vi "Color Frame Data FGV.vi"(6 "Command":enum16{"Get", "Initialize"}(ring), 8 "error in (no error)":errorcluster, 10 "FrameDescription":T1) -> (0 "error out":errorcluster, 2 "Byte Array":u8[](array[numeric]))   [LabVIEW 2014]
uses:
  controls/FrameDescription.ctl
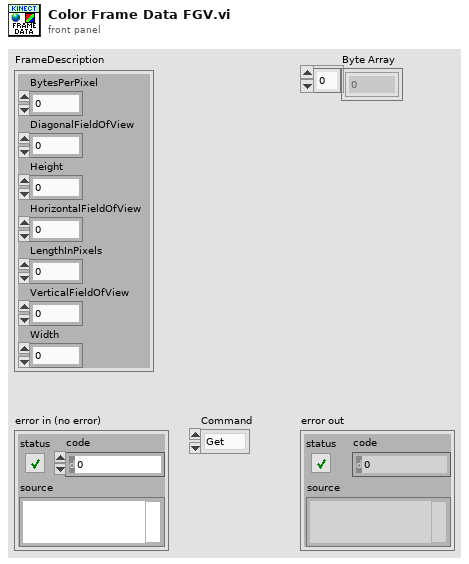
[diagram p1: front panel]
types:
  T1 = typedef "FrameDescription.ctl" = cluster{"BytesPerPixel":u32, "DiagonalFieldOfView":sgl, "Height":i32, "HorizontalFieldOfView":sgl, "LengthInPixels":u32, "VerticalFieldOfView":sgl, "Width":i32}
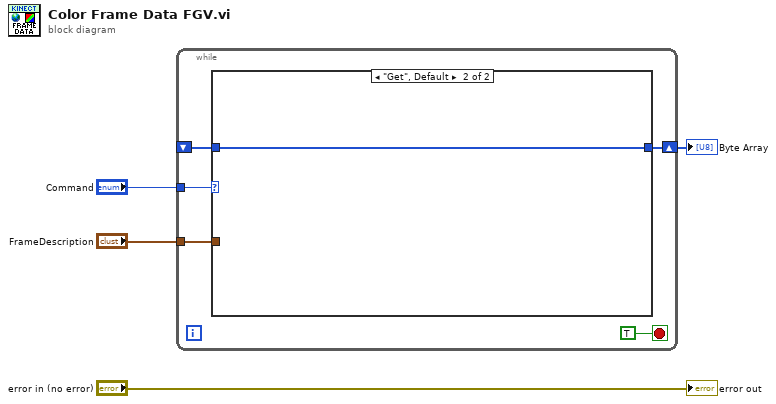
[diagram p0: block diagram]
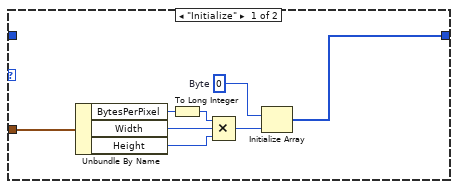
[diagram p2: hidden frame]
diagram:
  n1 = while {
    tunnel: "Command" -> [w9]
    tunnel: "FrameDescription" -> [w8]
    shift-right: [w7] -> w2
    shift-left: _ -> [w6]
    stop <- TRUE stop-if-true
    n2 = case shown="\"Get\", Default" w9 {
      tunnel: w8 -> [w15 _]
      tunnel: [w10 w18] -> w7
      tunnel: w6 -> [_ w18]
      frame "Initialize" {
        w16 = u8 0  # Byte
        n3 = Unbundle By Name(w15) -> ("BytesPerPixel"=w12:u32, "Width"=w14:i32, "Height"=w13:i32)
        n4 = To Long Integer(number=w12) -> (32bit integer=w11:i32)
        n5 = Compound Arithmetic op=MULTIPLY(w11, w14, w13) -> (w17:i32)
        n6 = Initialize Array(w16, w17) -> (w10:u8[])
      }
      frame "Get", Default {
      }
    }
  }
  "Byte Array" <- w2
  "error out" <- "error in (no error)"
